vi "AlliGator Apply Fit Result Constraints.vi"(8 "error in (no error)":errorcluster, 11 "AlliGator IV DVR in":refnum<data-value>) -> (0 "error out":errorcluster, 1 "Message":string, 3 "AlliGator IV DVR out":refnum<data-value>)   [LabVIEW 2021, in "AlliGator Decay Fit Parameter Map.lvlib"]
uses:
  AlliGator Decay Fit Parameter Map.lvlib
  Internal Variables/AlliGator Internal Variables v2.ctl
  <vilib>/vision/Image Controls.llb/IMAQ Image.ctl
  Internal Variables/AlliGator Gate Image Set.ctl
  Files/AlliGator FLI Dataset Type.ctl
  Files/AlliGator Data Series Type.ctl
  Dual-Channel Datasets/AlliGator Dataset Channel.ctl
  Settings/AlliGator Gate Arithmetic.ctl
  Source Image/AlliGator Displayed Image.ctl
  Image/Named ROI Description.ctl
  Phasor Graph/AlliGator Decay Metadata v3.ctl
  Decay Analysis/Decay Preprocessing/AlliGator Decay Background Subtraction Info.ctl
  Decay Analysis/Decay Preprocessing/AlliGator Baseline Subtraction Method.ctl
  Graphs/XY Graph/XY Graph Plot Shift Parameters.ctl
  Graphs/XY Graph/XY Graph Plot Shift Method.ctl
  Decay Analysis/Decay Preprocessing/AlliGator Decay Extrapolation Parameters.ctl
  Phasor/Calibration Phasor (m, phi).ctl
  Phasor/Phasor Reference Series.ctl
  Phasor/Phasor Calibration Map v2.ctl
  Phasor/Phasor (g, s).ctl
  Phasor Graph/AlliGator Raw Phasor Plot Data v5.ctl
  Phasor/Phasor Standard Deviation Options.ctl
  Phasor Plot/AlliGator Phasor Multi-Harmonic Data.ctl
  Phasor/Phasor Harmonic Data.ctl
  AlliGator Decay Fit Options & Parameters v4.ctl
  Fits/IRF(X)PSED/Decay Fit Options v4.ctl
  Fits/Decay Convolution/Decay Model.ctl
  Fits/Residual Type.ctl
  Fits/IRF(X)PSED/Fit Weights Type v2.ctl
  Fits/Non-linear Fitting Method v2.ctl
  Fits/Fit Calculation Method.ctl
  Fits/Non-linear Fitting Algorithm.ctl
  Decay Analysis/Decay Fit/AlliGator Decay Fit Parameter Constraints 2.ctl
  Fits/IRF(X)PSED/Decay Fit Parameters In List.ctl
  Fits/IRF(X)PSED/MLE Baseline Offset Type.ctl
  Decay Analysis/Decay Preprocessing/AlliGator Decay Preprocessing Parameters.ctl
  Fits/IRF(X)PSED/Decay Fit Parameters & Derived Quantities List v2.ctl
  Fits/IRF(X)PSED/Decay Fit Result Constraint.ctl
  AlliGator Parameter Maps Data.ctl
  Globals, Variables, Constants/AlliGator Variables List.ctl
  Variant/Variant to Data/Variant to Boolean.vi
  Variant/Variant to Data/Variant to U16.vi
  Globals, Variables, Constants/AlliGator Globals, Variables & Constants.lvlib
  Variant/Variant to Data/Variant to Data.lvlib
  Fits/Fits.lvlib
  Decay Analysis/Decay Preprocessing/AlliGator Decay Preprocessing.lvlib
  Decay Analysis/Decay Processing/AlliGator Decay Processing.lvlib
  Local Decay Window/AlliGator Local Decay Window.lvlib
  Utilities/Utilities.lvlib
  Phasor/Phasor.lvlib
  Image/Image.lvlib
  Phasor Graph/AlliGator Phasor Graph.lvlib
  Files/AlliGator Files.lvlib
  Internal Variables/AlliGator Internal Variables.lvlib
  Phasor Plot/AlliGator Phasor Plot.lvlib
  Source Image/AlliGator Source Image.lvlib
  Decay Analysis/Decay Fit/AlliGator Decay Fit.lvlib
  Settings/AlliGator Settings.lvlib
  Dual-Channel Datasets/AlliGator Dual-Channel Datasets.lvlib
  Graphs/XY Graph/XY Graph Add-Ons.lvlib
panel:
  # "see the License on the block diagram (Ctrl+E or Window:Show Block Diagram)"
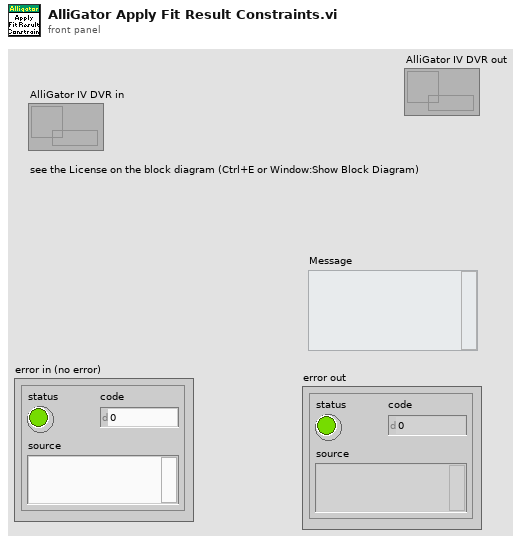
[diagram p1: front panel]
types:
  T1 = typedef "AlliGator Globals, Variables & Constants.lvlib/AlliGator Variables List.ctl" = enum16{"---- GUI ----", "GUI:Initialization Status", "GUI:State Indicators Refnum", "GUI:Original AlliGator Menu Items", "GUI:Current Action Loop State", "GUI:Script in progress", "GUI:Playback", "GUI:Loop Playback", "GUI:Search ROI Used", "GUI:Search ROI", "Decay Graph Max Legend Size", "Intensity Graph Max Legend Size", "Decay Statistics Graph Max Legend Size", "Phasor Graph Max Legend Size", "Phasor Ratio Graph Max Legend Size", "Lifetime Graph Max Legend Size", "---- Files ----", "Files:Export Dataset Frames as Individual Files", "Files:Show Batch Export Help Balloons", "Files:Frames in Dataset", "Files:ptu File Frame Start Indices", "Files:Current Frame in Dataset", "Files:Current Frame Timestamp", "Files:Dataset Loaded", "Files:Dataset Metadata", "Files:Dataset Channel", "Files:Dataset Data Description", "Files:Background Dataset Metadata", "Files:Background Dataset Channel", "Files:Background Dataset Data Description", "Files:Background File Subtraction", "Files:Background File Path", "Files:Background File Pile-up Correction", "Files:Background File Pixel Well Capacity", "Files:Background File Scaling Factor", "Files:Current Dataset Load Settings", "Files:Dataset Path", "Files:ICCD-specific Information", "Files:Macrotime Gate Separation", "------ Python Plugins ------", "Python Plugins:Information", "Python Plugins:Python Session", "Python Plugins:Valid Python Session?", "---- Source Image ----", "Source Image:ROIs", "Source Image:Current ROI", "Source Image:ROI Event Refnum", "X_Source Image:Display Range", "X_Source Image:Palette Information", "X_Source Image:Type of Displayed Image", "X_Time Gate Slider", "Source Image:Palette List", "Source Image:Scale", "Source Image:ROI Overlay Color", "Source Image:Overlay to Erase", "Source Image:Is Displayed Image Accumulated", "Source Image:White Light Image Modified", "Source Image:Mask Image Modified", "---- Image Profile Window ----", "Image Profile:Window Event Refnum", "Image Profile:IntensityType", "Image Profile:Intensity Average Type", "Image Profile:Intensity-weighted SDV", "Image Profile:Box Profile Type", "Image Profile:Window Open", "Image Profile:Plotted Fit Parameter", "------ Phasor Graph -------", "Phasor Graph:Show Line", "---- Phasor Plot ---", "Phasor Plot:Parameters Changed", "Phasor Plot:FLI Dataset Modified since last Calculation", "Phasor Harmonics Data", "Selected Phasor Harmonics", "Phasor Harmonic Manager Event Refnum", "Phasor Plot:ROIs", "Phasor Plot:Current ROI", "Phasor Plot:ROI Event Refnum", "Phasor Plot:Image Reference Points", "Phasor Plot:Computed", "Phasor Plot:Palette Information", "Phasor Plot:Palette List", "Phasor Plot:Phasor Ratio Palette Information", "Phasor Plot:Phasor Ratio Palette List", "Phasor Plot:Image Scale", "Phasor Plot:Image Overlay to Erase", "Phasor Plot:Image Elements to Update", "Phasor Plot:Current Calculation Parameters", "Phasor Plot:Current Calibration Options", "Phasor Plot:Reset Cumulated Phasor Plot", "Phasor Plot:Reference 1", "Phasor Plot:Lifetime Reference 1", "Phasor Plot:Reference 1 Frequency", "Phasor Plot:Reference 2", "Phasor Plot:Lifetime Reference 2", "Phasor Plot:Reference 2 Frequency", "---- Decay Analysis ----", "Number of Selected Decays to Fit", "LS Fit Results", "LAR Fit Results", "BS Fit Results", "Last Decay Max - Min", "Best Fit Parameters", "Best Fit Parameter Names", "Actual Size X", "Actual Size Y", "Binning X", "Binning Y", "Actual # Gates", "Dataset Number", "Gates to...", "Gates Skipped", "Gates to keep", "Gate Step", "Gate Separation", "Reversed Gates", "Pile-up Correction", "Pixel Well Capacity", "Background Subtracted", "Background Subtraction Method", "Background Definition Range", "Background File (deprecated)", "Number of Dataset Accumulated", "Array of Accumulated Dataset Paths", "Do Averaged Datasets", "Destination File Path", "Process Plot Target", "Use 1/D as Phasor Frequency", "---- Decay Fit Parameter Map -----", "Decay Fit Parameter Map:Palette Information", "Decay Fit Parameter Map:Palette List", "Decay Fit Parameter Map:X Resolution", "Decay Fit Parameter Map:Y Resolution", "Decay Fit Parameter Map:Use Decay Fit Result Constraints", "Decay Fit Parameter Map:Decay Fit Result Constraints", "Decay Fit Parameter Map:Decay Fit Result Constraints Applied", "---- Parameter Map ----", "Parameter Map:Palette Information", "Parameter Map:Palette List", "------- Local Decay Window ---------", "Local Decay Graph Window:Event Refnum", "Local Decay Graph Window:Use normalized IRF for convolution", "----- Miscellaneous ----", "Misc:Skippable Dialog Windows Status"}
  T2 = typedef "Fits.lvlib/Decay Fit Result Constraint.ctl" = cluster{"Fit Parameter":enum16{"Offset", "Baseline", "A_1", "tau_1", "A_2", "tau_2", "<tau>_a", "f1_a", "f2_a", "<tau>_i", "f1_i", "f2_i", "-", "R^2", "Chi^2", "Max Relative Residual", "<Residual ACF>", "Residual ACF SDV", "tau_2/tau_1"}, "Min Value":dbl, "Max Value":dbl, "Use Constraint":bool}
  T3 = typedef "IMAQ Image.ctl" = refnum<image>
  T4 = typedef "AlliGator Internal Variables.lvlib/AlliGator Internal Variables v2.ctl" = cluster{"----------------------------- Images -----------------------------":u8, "Displayed Image":T3, "White Light Image":T3, "Mask Image":T3, "ROI Mask Image":T3, "Current Dataset Images 1":T5, "Background Dataset Images 1":T5, "Current Dataset Images 2":T5, "Background Dataset Images 2":T5, "Current Dataset Arithmetic Images":T5, "Accumulated Dataset Images 1":T5, "Accumulated Dataset Images 2":T5, "Accumulated Dataset Arithmetic Images":T5, "----------------------------- File Paths -----------------------------":u8, "Phasor Plot Image":T3, "Decay Fit Parameter Map Image":T3, "Parameter Map Image":T3, "Single Data Point Path":path, "White Light Image Path":path, "Mask Image Path":path, "Time-Series Folder":path, "[Time-Series Paths]":path[], "----------------------------- FLI Dataset -----------------------------":u8, "Current Dataset":i32, "Single Dataset Type":T6, "Current Folder":string, "AlliGator Data Series Type":T7, "# Datasets":i32, "Dual-Channel Dataset":bool, "Selected Channel Name":string, "Dataset Channel":T8, "Channel Arithmetic":T9, "Dual-Channel Background Dataset":bool, "Background Channel":T8, "Dual-Channel Accumulated Dataset":bool, "Start Time":dbl, "[Time-Series Timestamps]":dbl[], "[Intensity Corrections]":dbl[], "Time Series Script":bool, "Type of Displayed Image":T10, "Gate Image Slide":u16, "# Gates":i32, "ROIs":T11[], "----------------------------- Decays -----------------------------":u8, "ROI Decay":cluster{"t Array":dbl[], "I Array":dbl[]}, "Valid Decay":bool, "Decay  Metadata":T13, "Reference Decay Plot Name":string, "Reference Decay":cluster{"t Array":dbl[], "I Array":dbl[]}, "Decay Shift Plot":cluster{"Time Stamps":dbl[], "Decay Shifts":dbl[]}, "[Decays Max Values]":sgl[], "[Decays Min Values]":sgl[], "----------------------------- Calibration -----------------------------":u8, "Calibration Phasor":T19, "Calibration Phasor Series":T20, "Phasor Calibration Map":T21, "Calibration Map MD5 Digest":string, "----------------------------- Phasor Graph -----------------------------":u8, "Last Raw Phasor":T22, "Last Calibrated Phasor":T22, "Last Calibrated Phasor SDV":T22, "Phasor Graph:Phasor Plot":cluster{"g Array":dbl[], "s Array":dbl[]}, "Phasor Graph:Phasor SDV Plot":cluster{"g Array":dbl[], "s Array":dbl[]}, "[Phasor Graph:Raw Phasor Plots]":T23[], "Phasor Plot locked to Ref 1":i32, "[Phasor Plot(s) locked to Ref 1]":i32[], "[Phasor Plot(s) locked to Ref 2]":i32[], "[Pixel Phasors]":T22[], "----------------------------- Phasor Plot -----------------------------":u8, "[[Sum Image]]":dbl[][], "[[CSG Phasors]]":csg[][], "[[Valid Pixel?]]":bool[][], "[[Phasor Ratios]]":dbl[][], "[[Average Lifetimes]]":dbl[][], "Amplitude Weighted Average Lifetime":bool, "I/m/phi Dataset":cluster{"I/m/phi Dataset?":bool, "Base Frequency":dbl[unit], "Harmonic Orders":u8[]}, "Multi Phasor Plot Data":T25, "----------------------------- Decay Fit Parameter Map -----------------------------":u8, "Decay Fit Options & Parameters":T27, "Fit Options: Decay Preprocessing Parameters":T38, "Fit Options: Reference Decay":cluster{"t Array":dbl[], "I Array":dbl[]}, "Is Full Image Parameters Map":bool, "Is Single-Pixels Parameters Map":bool, "NLSF Parameters Map X Resolution":i32, "NLSF Parameters Map Y Resolution":i32, "[Single Decay Fit Parameters]":dbl[], "Fit Model":T29, "[[Multiple Decays Fit Parameters]]":dbl[][], "[[Multiple Decays Fit Parameter SDVs]]":dbl[][], "[[IRFs]]":dbl[][], "[ROI Descriptors]":T12[], "IRF Array Time Axis":dbl[], "Decay Array Time Axis":dbl[], "[Decay Fit Parameter Names]":T39[], "[Decay Sum]":dbl[], "Array of Decay Fit Result Constraints":T2[], "Selected ROIs Array":bool[], "----------------------------- Parameter Maps -----------------------------":u8, "[Map Set Names]":string[], "[Parameter Maps]":T40[], "[[User-defined Quantities]]":dbl[][], "User-defined Quantity":string}
  T5 = typedef "AlliGator Internal Variables.lvlib/AlliGator Gate Image Set.ctl" = cluster{"SGL Gate Images":T3[], "SGL Sum Image":T3, "SGL Max Image":T3, "SGL Min Image":T3}
  T6 = typedef "AlliGator Files.lvlib/AlliGator FLI Dataset Type.ctl" = enum16{"HDF5 FLI Dataset", "Gate Image Folder", ".sdt FLI Dataset (Becker & Hickl)", ".ptu FLI Dataset (PicoQuant)", "SS1 FLI Dataset", "SS2 FLI Dataset", "I/m/phi Dataset", ".bin FLI Dataset (PicoQuant Binned)", ".bin FLI Dataset (Piccolo Binned)", ".mat FLI Dataset"}
  T7 = typedef "AlliGator Files.lvlib/AlliGator Data Series Type.ctl" = enum16{"Not a Supported Series", "Gate Images Folder Series", "SwissSPAD 2 Dataset Series", "B&H FLI Dataset Series", "PicoQuant PTU FLI Dataset Series", "PicoQuant BIN FLI Dataset Series", "Piccolo hist BIN FLI Dataset Series", "HDF5 FLI Dataset Series"}
  T8 = typedef "AlliGator Dual-Channel Datasets.lvlib/AlliGator Dataset Channel.ctl" = enum16{"G2", "INT"}
  T9 = typedef "AlliGator Settings.lvlib/AlliGator Gate Arithmetic.ctl" = enum16{"None", "INT-G2", "G2/INT*<INT>", "(1 - G2/INT)*<INT>"}
  T10 = typedef "AlliGator Source Image.lvlib/AlliGator Displayed Image.ctl" = enum16{"Single Gate", "Sum of All Gates", "Max of All Gates", "Min of All Gates", "-", "White Ligth Image", "Mask Image"}
  T11 = typedef "Image.lvlib/Named ROI Description.ctl" = cluster{"ROI Descriptor":T12, "ROI Name":string, "Overlay Color":u32}
  T12 = typedef "ROI Descriptor" = cluster{"Global Rectangle":i32[], "Contours":cluster{"ID":enum32{"External", "Internal"}, "Type":u32, "Coordinates":i32[]}[]}
  T13 = typedef "AlliGator Phasor Graph.lvlib/AlliGator Decay Metadata v3.ctl" = cluster{"ROI Descriptor":T12, "ROI Center":cluster{"X":i32, "Y":i32}, "Decay Background Subtraction Info":T14, "Decay Reverted":bool, "Decay Smoothened":bool, "Decay Straightened":bool, "Fitted Tau (Decay Straightening)":dbl, "Decay Shift Parameters":T16, "Decay Shifted":bool, "Decay Extrapolated":bool, "Decay Extrapolation Parameters":T18, "Decay Normalized":bool, "Fold Decay":bool, "# Folds":u32}
  T14 = typedef "AlliGator Decay Preprocessing.lvlib/AlliGator Decay Background Subtraction Info.ctl" = cluster{"Laser Period":dbl[unit], "Gate Duration":dbl[unit], "Baseline Subtraction Method":T15, "Background Definition Range":cluster{"Min Gate":dbl[unit], "Max Gate":dbl[unit]}, "Total Intensity w/o Bkgd Subtraction":dbl, "Bkgd-subtracted Intensity (exp)":dbl, "# Data Points":i32, "Background/Gate":dbl, "Fitted Lifetime":dbl[unit], "Bkgd-subtracted Intensity (theo)":dbl}
  T15 = typedef "AlliGator Decay Preprocessing.lvlib/AlliGator Baseline Subtraction Method.ctl" = enum16{"Mean", "Min", "Square Gated Single-Exponential", "File", "Constant"}
  T16 = typedef "XY Graph Add-Ons.lvlib/XY Graph Plot Shift Parameters.ctl" = cluster{"Type":T17, "Shift":dbl[unit], "Threshold":dbl, "Rotate":bool}
  T17 = typedef "XY Graph Add-Ons.lvlib/XY Graph Plot Shift Method.ctl" = enum16{"Default", "CFD", "Threshold", "Cross-Correlation"}
  T18 = typedef "AlliGator Decay Preprocessing.lvlib/AlliGator Decay Extrapolation Parameters.ctl" = cluster{"Additional Points":u32, "Head Fraction":dbl, "Fitted Tau":dbl, "Use Periodicity":bool, "Use Cursors":bool, "Tail Fraction":dbl}
  T19 = typedef "Phasor.lvlib/Calibration Phasor (m, phi).ctl" = cluster{"m":dbl, "phi":dbl, "Phasor Frequency":dbl[unit], "Reference Lifetime":dbl[unit]}
  T20 = typedef "Phasor.lvlib/Phasor Reference Series.ctl" = cluster{"m Array":dbl[], "phi Array":dbl[], "Phasor Frequency":dbl[unit], "Calibration Lifetime":dbl[unit]}
  T21 = typedef "Phasor.lvlib/Phasor Calibration Map v2.ctl" = cluster{"Phasor Frequency":dbl[unit], "Calibration Lifetime":dbl[unit], "ROI Centers":cluster{"X":i32, "Y":i32}[], "ROI Descriptors":T12[], "Map Resolution X":i32, "Map Resolution Y":i32, "z Array":cdb[]}
  T22 = typedef "Phasor.lvlib/Phasor (g, s).ctl" = cluster{"g":dbl, "s":dbl}
  T23 = typedef "AlliGator Phasor Graph.lvlib/AlliGator Raw Phasor Plot Data v5.ctl" = cluster{"Phasor Plot Name":string, "Raw Phasor Plot":T22[], "Phasor Frequency":dbl[unit], "[Decay Metadata]":T13[], "Raw Phasor Plot SDV":T22[], "Phasor SDV Options":T24, "[Calibration Phasor]":T19[], "Intensity Array":dbl[]}
  T24 = typedef "Phasor.lvlib/Phasor Standard Deviation Options.ctl" = cluster{"Compute Estimated SDV":bool, "# Replicas":u32, "Use Estimated Average Phasor":bool}
  T25 = typedef "AlliGator Phasor Plot.lvlib/AlliGator Phasor Multi-Harmonic Data.ctl" = cluster{"Base Frequency":dbl[unit], "# Harmonics":u8, "Harmonic Orders":u8[], "Phasor Plot Settings Checksum":u64, "Phasor Harmonic Data Array":T26[]}
  T26 = typedef "Phasor.lvlib/Phasor Harmonic Data.ctl" = cluster{"Phasor Harmonic Name":string, "Phasor Plot Settings Checksum":u64, "Phasor Frequency":dbl[unit], "Base Frequency":dbl[unit], "Harmonic Order":u8, "Phasor Plot Parameters":string, "Phasor Array [[CSG]]":csg[][], "Dataset File Path":path}
  T27 = typedef "AlliGator Decay Fit Parameter Map.lvlib/AlliGator Decay Fit Options & Parameters v4.ctl" = cluster{"SYNC Period":dbl[unit], "Fit Options":T28, "Fit Parameter Constraints":T35[], "MLE Baseline Offset":dbl, "MLE Baseline Offset Type":T37}
  T28 = typedef "Fits.lvlib/Decay Fit Options v4.ctl" = cluster{"Show Fit Residuals":bool, "Fit Model":T29, "Residual Type":T30, "Max Decay Percentile":dbl, "Min Decay Percentile":dbl, "Show Full Decay":bool, "Weights":T31, "Fitting Method":T32, "Compute Parameter Uncertainties":bool, "Periodic Boundaries":bool, "Model Calculation":T33, "Period":dbl[unit], "Termination Criteria":cluster{"Max Iterations":i32, "Max Function Calls":i32, "Max Time":dbl[unit], "Function Tolerance":dbl, "Parameter Tolerance":dbl, "Gradient Tolerance":dbl, "Min Lambda":dbl, "Max Lambda":dbl, "Initial Tick Count":u32}, "Offset Resolution":dbl[unit], "Use Local IRF":bool, "Fitting Algorithm":T34, "Show Confidence Interval ":bool, "Confidence Level":dbl}
  T29 = typedef "Fits.lvlib/Decay Model.ctl" = enum16{"1-Exponential", "2-Exponentials"}
  T30 = typedef "Fits.lvlib/Residual Type.ctl" = enum16{"Standard", "Normalized", "Reduced"}
  T31 = typedef "Fits.lvlib/Fit Weights Type v2.ctl" = enum16{"Unweighted", "1/Variance (Neyman)", "1/Variance (Pearson)", "Best of All"}
  T32 = typedef "Fits.lvlib/Non-linear Fitting Method v2.ctl" = enum16{"Least Square", "Least Absolute Residual", "Bisquare", "MLE", "-", "Best of All"}
  T33 = typedef "Fits.lvlib/Fit Calculation Method.ctl" = enum16{"Simulation", "Convolution", "Integration"}
  T34 = typedef "Fits.lvlib/Non-linear Fitting Algorithm.ctl" = enum16{"Levenberg-Marquardt", "Trust-Region Dogleg"}
  T35 = typedef "AlliGator Decay Fit.lvlib/AlliGator Decay Fit Parameter Constraints 2.ctl" = cluster{"Fit Parameter":T36, "Min Value":dbl, "Max Value":dbl, "Global":bool, "Used":bool}
  T36 = typedef "Fits.lvlib/Decay Fit Parameters In List.ctl" = enum16{"Offset", "Baseline", "A_1", "tau_1", "A_2", "tau_2"}
  T37 = typedef "Fits.lvlib/MLE Baseline Offset Type.ctl" = enum32{"Absolute", "Percentage"}
  T38 = typedef "AlliGator Decay Preprocessing.lvlib/AlliGator Decay Preprocessing Parameters.ctl" = cluster{"Background Subtraction":bool, "Straighten Decay":bool, "Reverse Gates":bool, "1-Normalized Decay":bool, "Smoothen Decay":bool, "Smoothing Parameter":dbl, "Shift Decay":bool, "Decay Shift Parameters":T16, "Extrapolate Decay":bool, "Additional Points":u32, "Head Fraction":dbl, "Pixel-Normalize Decay":bool, "Use Periodicity":bool, "Use Cursors":bool, "Tail Fraction":dbl, "Use Decay Pre-Processing":bool, "Fold Decay":bool, "# Folds":u32, "[0-1]-Normalized Decay":bool}
  T39 = typedef "Fits.lvlib/Decay Fit Parameters & Derived Quantities List v2.ctl" = enum16{"Offset", "Baseline", "A_1", "tau_1", "A_2", "tau_2", "<tau>_a", "f1_a", "f2_a", "<tau>_i", "f1_i", "f2_i", "-", "R^2", "Chi^2"}
  T40 = typedef "AlliGator Decay Fit Parameter Map.lvlib/AlliGator Parameter Maps Data.ctl" = cluster{"Map Set Name":string, "[Parameter Names]":string[], "[[Parameters]]":dbl[][], "[[Parameter SDVs]]":dbl[][], "Decay Array Time Axis":dbl[], "[[IRFs]]":dbl[][], "IRF Array Time Axis":dbl[], "X Resolution":i32, "Y Resolution":i32, "Intensity Array":dbl[]}
  T41 = cluster{"t Axis":dbl[], "ROI Intensity Array":dbl[]}
  T42 = cluster{"IRF Array Time Axis":dbl[], "[[IRFs]]":dbl[]}
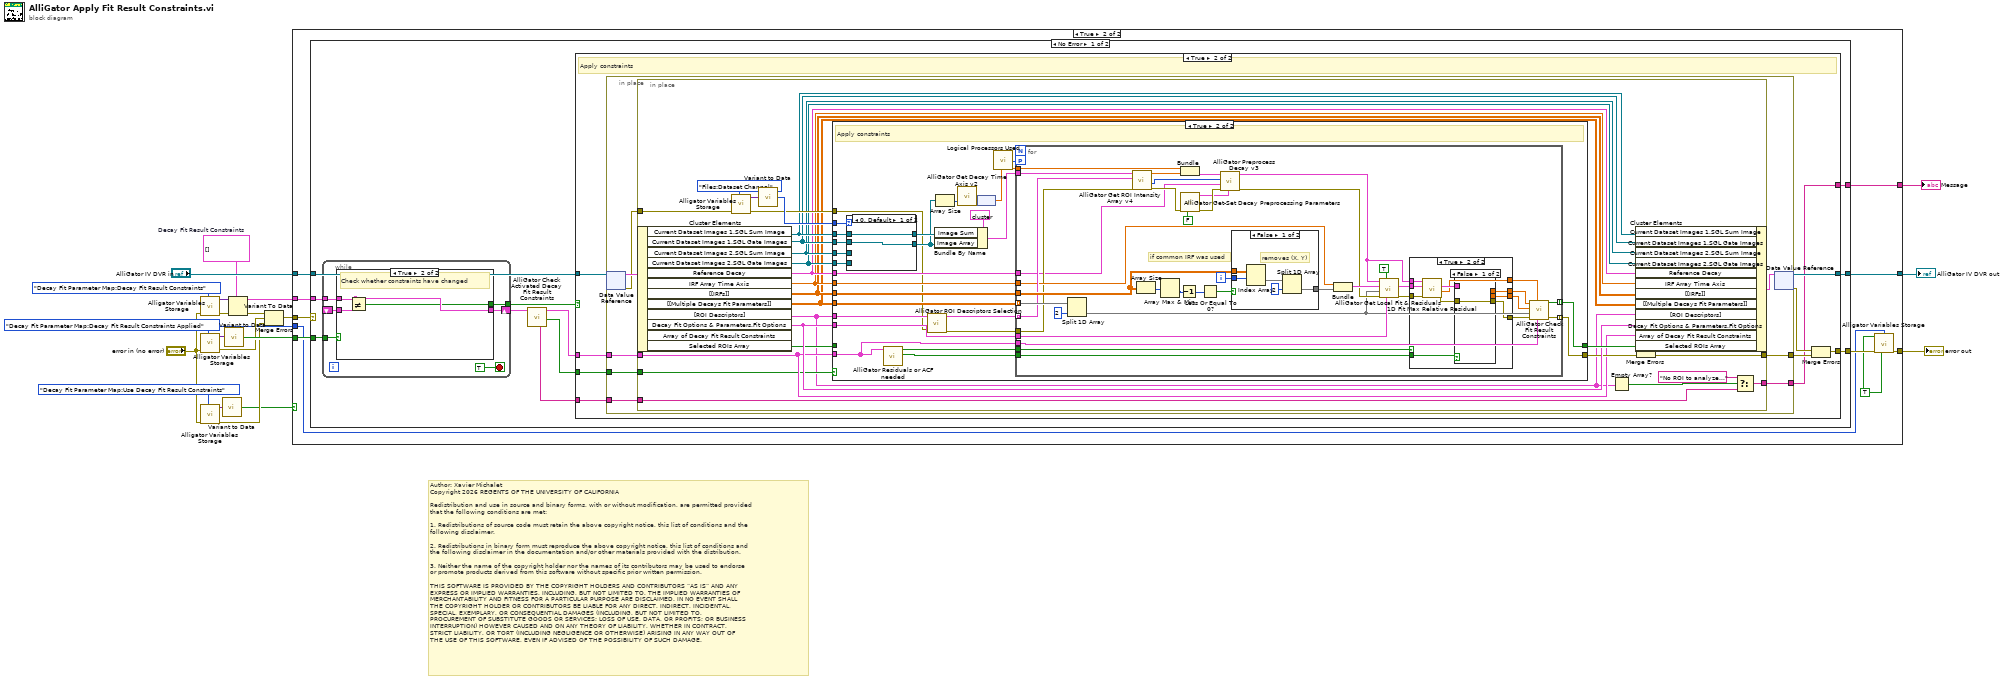
[diagram p0: block diagram]
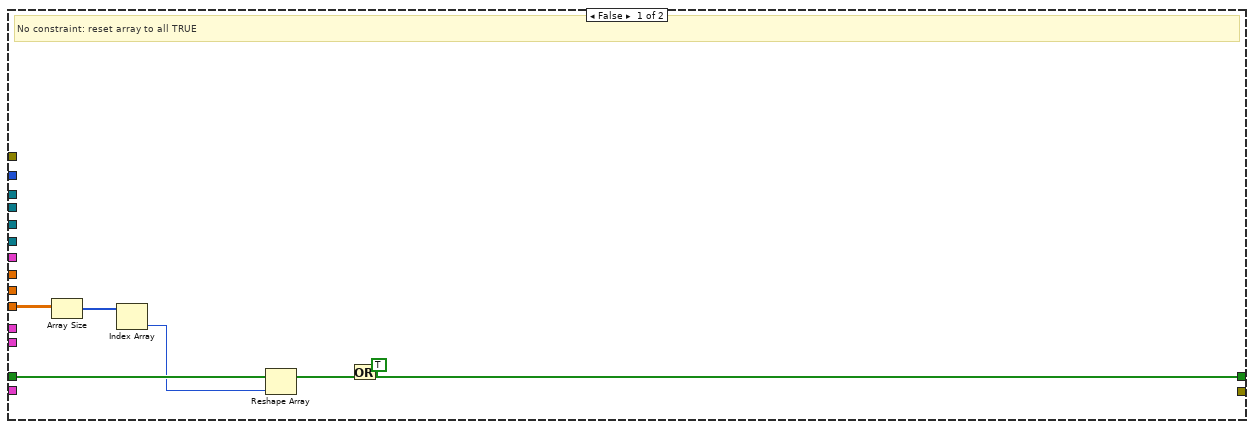
[diagram p4: hidden frame]
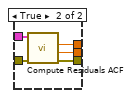
[diagram p6: hidden frame]
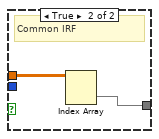
[diagram p7: hidden frame]
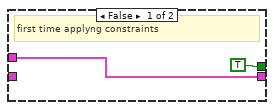
[diagram p9: hidden frame]
diagram:
  w13 = T2[] []  # Decay Fit Result Constraints
  w7 = AlliGator_Variables_List."Decay Fit Parameter Map:Decay Fit Result Constraints Applied" ("Alligator Variable")
  # "Author: Xavier Michalet\nCopyright 2026 REGENTS OF THE UNIVERSITY OF CALIFORNIA\n\nRedistribution and use in source and binary forms, with or without modification, are permitted provided\nthat the following conditions are met:\n\n1. Redistributions of source code must retain the above copyright notice, this list of conditions and the\nfollowing disclaimer.\n\n2. Redistributions in binary form must reproduce the above copyright notice, this list of conditions and\nthe following disclaimer in the documentation and/or other materials provided with the distribution.\n\n3. Neither the name of the copyright holder nor the names of its contributors may be used to endorse \nor promote products derived from this software without specific prior written permission.\n\nTHIS SOFTWARE IS PROVIDED BY THE COPYRIGHT HOLDERS AND CONTRIBUTORS “AS IS” AND ANY \nEXPRESS OR IMPLIED WARRANTIES, INCLUDING, BUT NOT LIMITED TO, THE IMPLIED WARRANTIES OF\nMERCHANTABILITY AND FITNESS FOR A PARTICULAR PURPOSE ARE DISCLAIMED. IN NO EVENT SHALL\nTHE COPYRIGHT HOLDER OR CONTRIBUTORS BE LIABLE FOR ANY DIRECT, INDIRECT, INCIDENTAL, \nSPECIAL, EXEMPLARY, OR CONSEQUENTIAL DAMAGES (INCLUDING, BUT NOT LIMITED TO, \nPROCUREMENT OF SUBSTITUTE GOODS OR SERVICES; LOSS OF USE, DATA, OR PROFITS; OR BUSINESS\nINTERRUPTION) HOWEVER CAUSED AND ON ANY THEORY OF LIABILITY, WHETHER IN CONTRACT, \nSTRICT LIABILITY, OR TORT (INCLUDING NEGLIGENCE OR OTHERWISE) ARISING IN ANY WAY OUT OF\nTHE USE OF THIS SOFTWARE, EVEN IF ADVISED OF THE POSSIBILITY OF SUCH DAMAGE."
  n1 = call "Alligator Variables Storage.vi"("AlliGator Variable"=AlliGator_Variables_List."Decay Fit Parameter Map:Decay Fit Result Constraints", "Error In"="error in (no error)") -> ("Error Out"=w14:errorcluster, "Data out"=w15:variant)  [unwired: 7 in, 1 out]
  n2 = call "Alligator Variables Storage.vi"("AlliGator Variable"=w7, "Error In"="error in (no error)") -> ("Error Out"=w10:errorcluster, "Data out"=w18:variant)  [unwired: 7 in, 1 out]
  n3 = call "Alligator Variables Storage.vi"("AlliGator Variable"=AlliGator_Variables_List."Decay Fit Parameter Map:Use Decay Fit Result Constraints", "Error In"="error in (no error)") -> ("Error Out"=w4:errorcluster, "Data out"=w3:variant)  [unwired: 7 in, 1 out]
  n4 = call-poly "Variant to Data.vi"("Variant"=w3) -> ("Value"=w2:bool)  [unwired: 8 in]
  n5 = call-poly "Variant to Data.vi"("Variant"=w18) -> ("Value"=w17:bool)  [unwired: 8 in]
  n6 = Variant To Data(error in=w14, type=w13, Variant=w15) -> (data=w12:T2[], error out=w11:errorcluster)
  n7 = Merge Errors(w11, w10, w4) -> (w9:errorcluster)
  n8 = case shown="True" w2 {
    tunnel: [w22 w32] -> w20
    tunnel: "AlliGator IV DVR in" -> [w22 w31]
    tunnel: w17 -> [_ w30]
    tunnel: w12 -> [_ w29]
    tunnel: w9 -> [w21 w28]
    tunnel: [w21 w26] -> w8
    tunnel: w7 -> [_ w24]
    tunnel: [_ w23] -> w1
    frame False {
    }
    frame True {
      w25 = TRUE ("Get(F)/Set")
      n9 = case shown="No Error" w28 {
        selector: w28 -> [_ w201]
        tunnel: [w43 w200] -> w32
        tunnel: w31 -> [w42 w200]
        tunnel: [w41 w201] -> w27
        tunnel: w30 -> [w40 _]
        tunnel: w29 -> [w38 _]
        tunnel: [w37 _] -> w23
        frame No Error {
          n10 = while {
            tunnel: w40 -> [w194]
            tunnel: w38 -> [w192]
            shift-right: [w191] -> w36
            shift-left: _ -> [w190]
            tunnel: [w189] -> w39
            stop <- TRUE stop-if-true
            n11 = case shown="True" w194 {
              tunnel: w192 -> [w196 w198]
              tunnel: [w196 w198] -> w191
              tunnel: w190 -> [_ w199]
              tunnel: [TRUE w197] -> w189
              frame False {
                # "first time applyng constraints"
              }
              frame True {
                # "Check whether constraints have changed"
                n12 = Not Equal?(x=w198, y=w199) -> (x != y?=w197:bool)
              }
            }
          }
          n13 = call "AlliGator Check Activated Decay Fit Result Constraints.vi"("Decay Fit Result Constraints"=w36) -> ("Any constraints?"=w35:bool, "Decay Fit Result Constraints (dup)"=w34:T2[], "Message"=w33:string)  [unwired: 8 in]
          n14 = case shown="True" w39 {
            tunnel: [w45 w54] -> w43
            tunnel: w42 -> [w45 w53]
            tunnel: [_ w51] -> w41
            tunnel: [w44 w46] -> w37
            tunnel: w35 -> [_ w49]
            tunnel: w34 -> [_ w48]
            tunnel: w33 -> [w44 w47]
            frame False {
              # "Constraints already applied and they haven't been modified"
            }
            frame True {
              # "Apply constraints"
              n15 = in-place {
                in-place-border: [w59] -> w50
                in-place-border: w49 -> [w58]
                in-place-border: w48 -> [w57]
                in-place-border: w47 -> [w56]
                in-place-border: [w55] -> w46
                n16 = in-place-dvr #1(w53) -> (w62:T4, w60:errorcluster)
                n17 = in-place {
                  in-place-border: w60 -> [w85]
                  in-place-border: [w71] -> w59
                  in-place-border: w57 -> [w70]
                  in-place-border: w58 -> [w69]
                  in-place-border: w56 -> [w65]
                  in-place-border: [w64] -> w55
                  n18 = in-place-cluster #2(w62) -> ("Current Dataset Images 1.SGL Sum Image"=w82:T3, "Current Dataset Images 1.SGL Gate Images"=w81:T3[], "Current Dataset Images 2.SGL Sum Image"=w80:T3, "Current Dataset Images 2.SGL Gate Images"=w79:T3[], "Reference Decay"=w78:cluster{"t Array":dbl[], "I Array":dbl[]}, "IRF Array Time Axis"=w77:dbl[], "[[IRFs]]"=w76:dbl[][], "[[Multiple Decays Fit Parameters]]"=w75:dbl[][], "[ROI Descriptors]"=w67:T12[], "Decay Fit Options & Parameters.Fit Options"=w73:T28, "Selected ROIs Array"=w68:bool[])  [unwired: 1 out]
                  n19 = call "Alligator Variables Storage.vi"("AlliGator Variable"=AlliGator_Variables_List."Files:Dataset Channel" ("Alligator Variable"), "Error In"=w85) -> ("Error Out"=w83:errorcluster, "Data out"=w86:variant)  [unwired: 7 in, 1 out]
                  n20 = call-poly "Variant to Data.vi"("Variant"=w86) -> ("U16 Value"=w84:u16)  [unwired: 8 in]
                  n21 = case shown="True" w69 {
                    tunnel: w67 -> [_ w121]
                    tunnel: w84 -> [_ w119]
                    tunnel: w83 -> [_ w100]
                    tunnel: w82 -> [_ w111]
                    tunnel: w81 -> [_ w110]
                    tunnel: w80 -> [_ w109]
                    tunnel: w79 -> [_ w108]
                    tunnel: w78 -> [_ w107]
                    tunnel: w77 -> [_ w106]
                    tunnel: w76 -> [_ w105]
                    tunnel: w75 -> [w94 w104]
                    tunnel: [w88 w103] -> w74
                    tunnel: w73 -> [_ w102]
                    tunnel: [_ w101] -> w72
                    tunnel: w70 -> [_ w97]
                    tunnel: w68 -> [w92 _]
                    frame False {
                      # "No constraint: reset array to all TRUE"
                      n22 = Array Size(array=w94) -> (size(s)=w93:i32[])
                      n23 = Index Array(array=w93) -> (element=w91:i32)  [unwired: 1 in]
                      n24 = Reshape Array(w92, w91) -> (w90:bool[])
                      n25 = Or(x=TRUE ("Selected"), y=w90) -> (x .or. y?=w88:bool[])
                    }
                    frame True {
                      # "Apply constraints"
                      n26 = case shown="0, Default" w119 {
                        tunnel: [w186 w188] -> w117
                        tunnel: w109 -> [_ w188]
                        tunnel: w108 -> [_ w187]
                        tunnel: [w185 w187] -> w112
                        tunnel: w111 -> [w186 _]
                        tunnel: w110 -> [w185 _]
                        frame 0, Default {
                        }
                        frame 1 {
                        }
                      }
                      n27 = call "AlliGator Residuals or ACF needed.vi"("Decay Fit Result Constraints"=w97) -> ("Compute ACF"=w95:bool, "Compute Residuals"=w96:bool)  [unwired: 9 in]
                      n28 = call "AlliGator ROI Descriptors Selection.vi"("Error In"=w100, "[ROI Descriptors]"=w121) -> ("Error Out"=w99:errorcluster, "[ROI Descriptors]"=w120:T12[])  [unwired: 7 in, 1 out]
                      n29 = Bundle By Name(cluster=cluster{"Image Sum":T3, "Image Array":T3[]} {"Image Sum"=refnum, "Image Array"=[]} ("Images"), "Image Sum"=w117, "Image Array"=w112) -> (w116:cluster{"Image Sum":T3, "Image Array":T3[]})
                      n30 = Array Size(array=w112) -> (size(s)=w114:i32)
                      n31 = call "AlliGator Get Decay Time Axis v2.vi"("Number of Gates"=w114) -> ("t Array"=w115:dbl[unit][])  [unwired: 14 in]
                      n32 = node(w115) -> (w113:dbl[])
                      n33 = call "Logical Processors Used.vi"() -> ("# Logical Processor Used"=w98:i32)  [unwired: 6 in]
                      n34 = for {
                        tunnel: w104 -> [w159] mode=indexing
                        tunnel: w105 -> [w153]
                        tunnel: w120 -> [w144] mode=indexing
                        tunnel: w116 -> [w145]
                        tunnel: w99 -> [w138]
                        tunnel: w113 -> [w143]
                        tunnel: w106 -> [w141]
                        tunnel: w107 -> [w137]
                        tunnel: w102 -> [w136]
                        tunnel: w97 -> [w135]
                        tunnel: [w131] -> w103 mode=indexing
                        tunnel: [w128] -> w101 mode=indexing
                        workers-P: w98 -> [_]
                        tunnel: w96 -> [w123]
                        tunnel: w95 -> [w122]
                        i -> [w154]
                        # "if common IRF was used"
                        n35 = Split 1D Array(array=w159, index=2) -> (second subarray=w134:dbl[])  [unwired: 1 out]
                        n36 = call "AlliGator Get ROI Intensity Array v4.vi"("error in (no error)"=w138, "ROI Descriptor"=w144, "Images"=w145) -> ("Error Out"=w152:errorcluster, "# Valid Pixels"=w150:i32, "ROI Intensity Array"=w146:dbl[])  [unwired: 3 in, 3 out]
                        n37 = Array Size(array=w153) -> (size(s)=w156:i32[])
                        n38 = Array Max & Min(array=w156) -> (min value=w157:i32)  [unwired: 3 out]
                        n39 = Decrement(x=w157) -> (x-1=w158:i32)
                        n40 = Bundle(w143, "ROI Intensity Array"=w146) -> (w149:cluster{dbl[], "ROI Intensity Array":dbl[]})  [unwired: 1 in]
                        n41 = call "AlliGator Get-Set Decay Preprocessing Parameters.vi"("Get (F)/Set"=FALSE, "Error In"=w152) -> ("Error Out"=w151:errorcluster, "Decay Preprocessing Parameters out"=w148:T38)  [unwired: 8 in]
                        n42 = Less Or Equal To 0?(x=w158) -> (x <= 0?=w155:bool)
                        n43 = call "AlliGator Preprocess Decay v3.vi"("Decay Preprocessing Parameters"=w148, "Error In"=w151, "Time-Gated Reference Decay"=w137, "# Pixels"=w150, "Decay (in)"=w149) -> ("Error Out"=w139:errorcluster, "Decay (out)"=w125:T41)  [unwired: 3 in, 2 out]
                        n44 = case shown="False" w155 {
                          tunnel: w153 -> [w182 w184]
                          tunnel: [w179 w183] -> w142
                          tunnel: w154 -> [w181 _]
                          frame False {
                            # "removes (X, Y)"
                            n45 = Index Array(array=w182, index (row)=w181) -> (element=w180:dbl[])  [unwired: 1 in]
                            n46 = Split 1D Array(array=w180, index=2) -> (second subarray=w179:dbl[])  [unwired: 1 out]
                          }
                          frame True {
                            # "Common IRF"
                            n47 = Index Array(array=w184) -> (element=w183:dbl[])  [unwired: 2 in]
                          }
                        }
                        n48 = Bundle("IRF Array Time Axis"=w141, "[[IRFs]]"=w142) -> (w140:T42)  [unwired: 1 in]
                        n49 = call "AlliGator Get Local Fit & Residuals.vi"("Fit Options"=w136, "Use Normalized IRF (T)"=TRUE, "Error In"=w139, "All Fit Parameters (w tau)"=w134, "IRF"=w140, "Decay Plot"=w125) -> ("Error Out"=w127:errorcluster, "Residual Plot"=w126:cluster{"X Array":dbl[], "Y Array":dbl[]})  [unwired: 2 in, 2 out]
                        n50 = case shown="True" w123 {
                          tunnel: [_ w171] -> w133
                          tunnel: [_ w170] -> w132
                          tunnel: [w161 w169] -> w129
                          tunnel: w127 -> [w161 w168]
                          tunnel: w126 -> [_ w166]
                          tunnel: w125 -> [_ w165]
                          tunnel: [_ w163] -> w124
                          tunnel: w122 -> [_ w162]
                          frame False {
                          }
                          frame True {
                            n51 = call "1D Fit Max Relative Residual.vi"("error in (no error)"=w168, "Residual Plot"=w166, "Plot"=w165) -> ("error out"=w167:errorcluster, "Max Relative Residual"=w163:dbl, "Residual Plot (dup)"=w164:cluster{"X Array":dbl[], "Y Array":dbl[]})  [unwired: 6 in]
                            n52 = case shown="False" w162 {
                              tunnel: [_ w177] -> w171
                              tunnel: [_ w176] -> w170
                              tunnel: [w172 w175] -> w169
                              tunnel: w167 -> [w172 w174]
                              tunnel: w164 -> [_ w173]
                              frame False {
                              }
                              frame True {
                                n53 = call "Compute Residuals ACF.vi"("Error In"=w174, "Residual Plot in"=w173) -> ("Error Out"=w175:errorcluster, "ACF SDV"=w176:dbl, "ACF Mean"=w177:dbl)  [unwired: 5 in, 2 out]
                              }
                            }
                          }
                        }
                        n54 = call "AlliGator Check Fit Result Constraints.vi"("Array of Decay Fit Result Constraints"=w135, "Max Relative Residual"=w124, "Error In"=w129, "Fit Parameters"=w134, "ACF SDV"=w132, "ACF Mean"=w133) -> ("Error Out"=w128:errorcluster, "Constraints Stisfied?"=w131:bool)  [unwired: 4 in]
                      }
                    }
                  }
                  n55 = Empty Array?(array=w67) -> (empty?=w66:bool)
                  n56 = in-place-cluster #2("Current Dataset Images 1.SGL Sum Image"=w82, "Current Dataset Images 1.SGL Gate Images"=w81, "Current Dataset Images 2.SGL Sum Image"=w80, "Current Dataset Images 2.SGL Gate Images"=w79, "Reference Decay"=w78, "IRF Array Time Axis"=w77, "[[IRFs]]"=w76, "[[Multiple Decays Fit Parameters]]"=w75, "[ROI Descriptors]"=w67, "Decay Fit Options & Parameters.Fit Options"=w73, "Array of Decay Fit Result Constraints"=w70, "Selected ROIs Array"=w74) -> (w61:T4)
                  n57 = Merge Errors(w72) -> (w71:errorcluster)
                  n58 = Select(t="No ROI to analyze...", s=w66, f=w65) -> (s? t:f=w64:string)
                }
                n59 = in-place-dvr #1(w61) -> (w54:refnum<data-value>, w52:errorcluster)
              }
              n60 = Merge Errors(w52, w50) -> (w51:errorcluster)
            }
          }
        }
        frame Error {
        }
      }
      n61 = call "Alligator Variables Storage.vi"("Get(F)/Set"=w25, "AlliGator Variable"=w24, "Error In"=w27, "Data in"=w25) -> ("Error Out"=w26:errorcluster)  [unwired: 5 in, 2 out]
    }
  }
  "error out" <- w8
  "AlliGator IV DVR out" <- w20
  "Message" <- w1
